vi "sub_statistics.vi"(7 "cmd":enum16{"ini", "read", "write"}(ring), 8 "error in":errorcluster) -> (0 "error out":errorcluster caption="error in")   [LabVIEW 2019]
uses:
  Ctrl/pid-in-params.ctl
  Ctrl/cmd_ini-RW.ctl
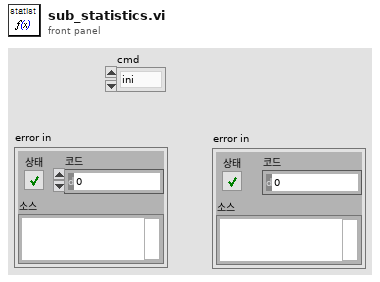
[diagram p1: front panel]
types:
  T1 = typedef "pid-in-params.ctl" = enum16{"read", "write"}
  T2 = typedef "cmd_ini-RW.ctl" = enum16{"ini", "read", "write"}
  T3 = cluster{"deg_agv-lookahead":dbl, "deg_waypoint":dbl, "deg_gap":dbl, "deg_target":dbl, "pid output":dbl, "dis-gap":dbl, "deg_agv-center":dbl}
  T4 = typedef "statistics_val.ctl" = cluster{"gap plus mean":dbl, "gap plus max":dbl, "gap plus sum":dbl, "gap minus mean":dbl, "gap minus max":dbl, "gap minus sum":dbl, "gap abs mean":dbl, "gap abs max":dbl, "gap abs sum":dbl, "wpt length":dbl, "total moving time":dbl, "average speed":dbl, "plus gap count":u64, "minus gap count":u64, "drive length":dbl}
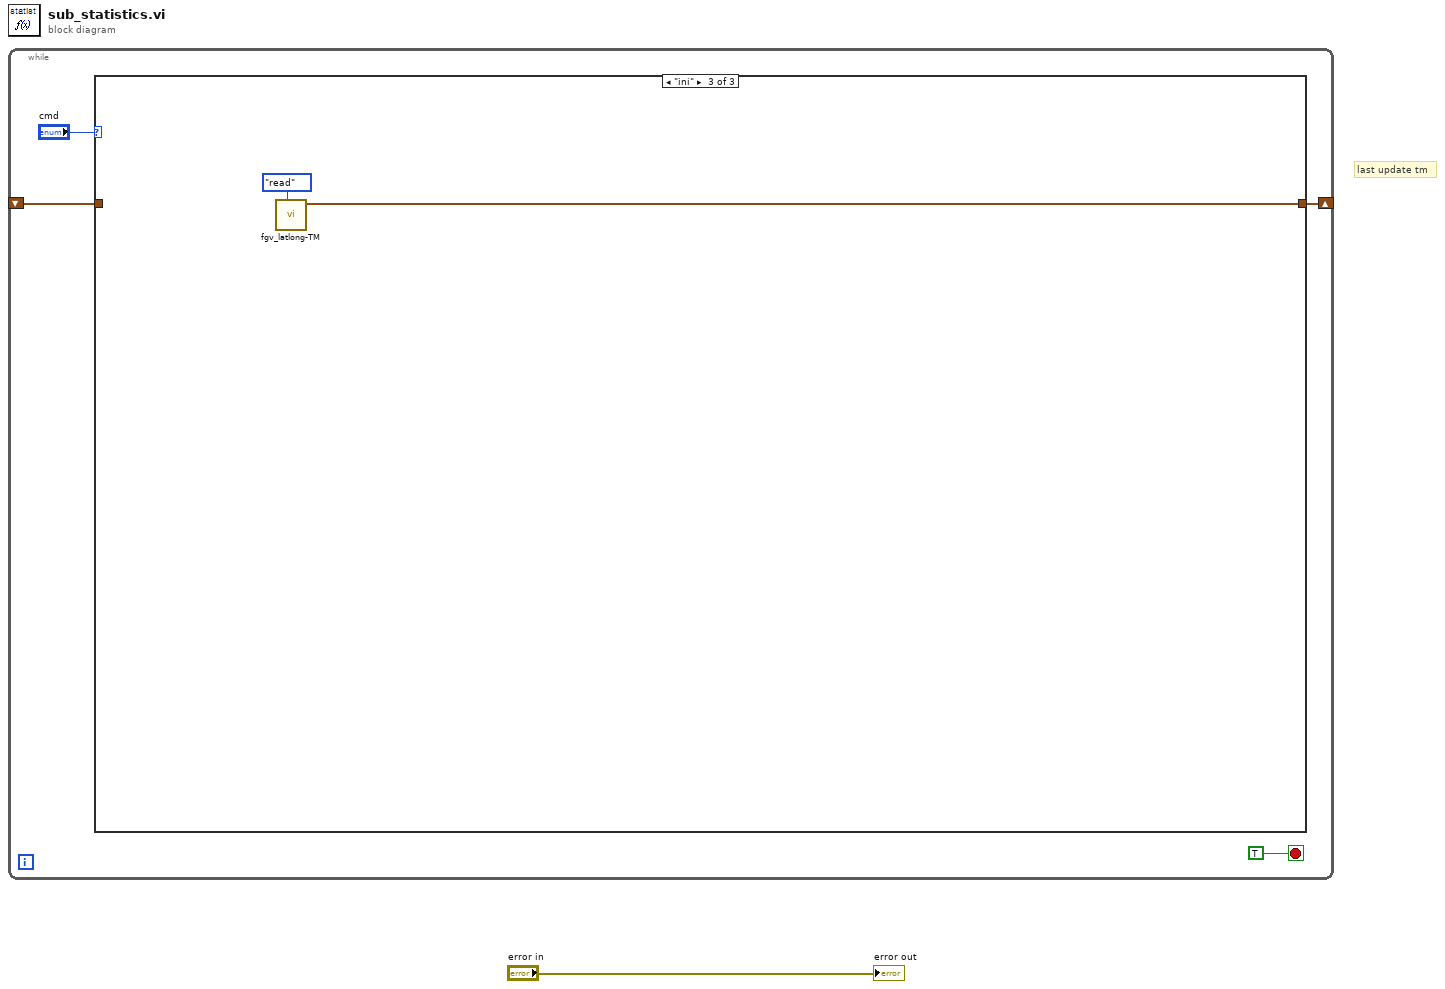
[diagram p0: block diagram]
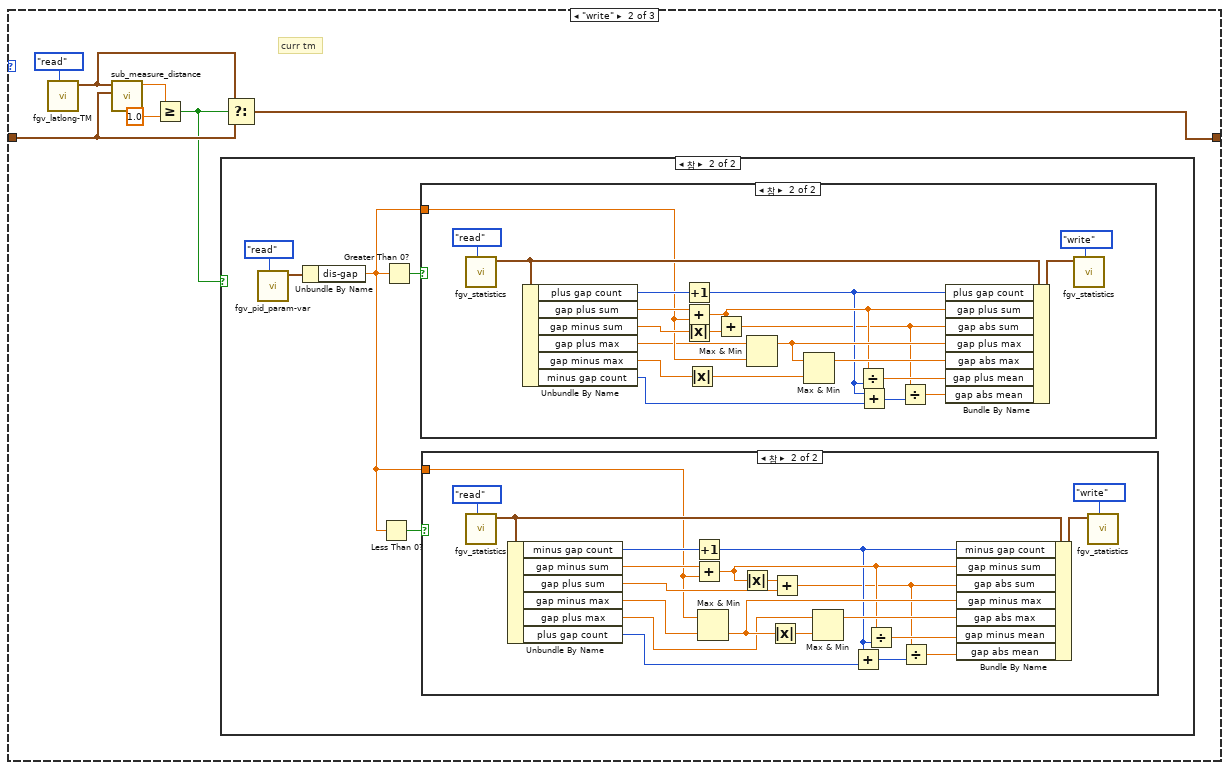
[diagram p3: hidden frame]
diagram:
  # "last update tm"
  n1 = while {
    shift-right: [w3] -> _
    shift-left: _ -> [w2]
    stop <- TRUE stop-if-true
    n2 = case shown="\"ini\"" "cmd" {
      tunnel: [w6 w8 w61] -> w3
      tunnel: w2 -> [w6 w9 _]
      frame "read", Default {
      }
      frame "write" {
        # "curr tm"
        n3 = call "fgv_latlong-TM.vi"("cmd"=enum16{"write", "read"}."read") -> ("tm out"=w10:cluster{dbl, dbl})  [unwired: 9 in, 1 out]
        n4 = call "sub_measure_distance.vi"("pt 2"=w9, "pt 1"=w10) -> ("distance"=w12:dbl)  [unwired: 9 in]
        n5 = Greater Or Equal?(x=w12, y=1.0) -> (x >= y?=w7:bool)
        n6 = case shown="참" w7 {
          frame False {
          }
          frame True {
            n7 = call "fgv_pid_param-var.vi"("cmd"=pid-in-params."read") -> ("pid-var_output"=w17:T3)  [unwired: 10 in]
            n8 = Unbundle By Name(w17) -> ("dis-gap"=w14:dbl)
            n9 = Less Than 0?(x=w14) -> (x < 0?=w15:bool)
            n10 = Greater Than 0?(x=w14) -> (x > 0?=w16:bool)
            n11 = case shown="참" w16 {
              tunnel: w14 -> [_ w52]
              frame False {
              }
              frame True {
                n12 = call "fgv_statistics.vi"("cmd"=cmd_ini-RW."read") -> ("statistics values out"=w59:T4)  [unwired: 10 in]
                n13 = Unbundle By Name(w59) -> ("plus gap count"=w58:u64, "gap plus sum"=w55:dbl, "gap minus sum"=w54:dbl, "gap plus max"=w51:dbl, "gap minus max"=w49:dbl, "minus gap count"=w44:u64)
                n14 = Increment(x=w58) -> (x+1=w43:u64)
                n15 = Add(x=w55, y=w52) -> (x+y=w45:dbl)
                n16 = Absolute Value(x=w54) -> (abs(x)=w53:dbl)
                n17 = Absolute Value(x=w49) -> (abs(x)=w48:dbl)
                n18 = Add(x=w45, y=w53) -> (x+y=w42:dbl)
                n19 = Max & Min(x=w51, y=w52) -> (max(x,y)=w50:dbl)  [unwired: 1 out]
                n20 = Max & Min(x=w50, y=w48) -> (max(x,y)=w47:dbl)  [unwired: 1 out]
                n21 = Divide(x=w45, y=w43) -> (x/y=w46:dbl)
                n22 = Add(x=w43, y=w44) -> (x+y=w41:u64)
                n23 = Divide(x=w42, y=w41) -> (x/y=w40:dbl)
                n24 = Bundle By Name(cluster=w59, "plus gap count"=w43, "gap plus sum"=w45, "gap abs sum"=w42, "gap plus max"=w50, "gap abs max"=w47, "gap plus mean"=w46, "gap abs mean"=w40) -> (w60:T4)
                n25 = call "fgv_statistics.vi"("cmd"=cmd_ini-RW."write", "statistics values"=w60) -> ()  [unwired: 9 in, 1 out]
              }
            }
            n26 = case shown="참" w15 {
              tunnel: w14 -> [_ w32]
              frame False {
              }
              frame True {
                n27 = call "fgv_statistics.vi"("cmd"=cmd_ini-RW."read") -> ("statistics values out"=w38:T4)  [unwired: 10 in]
                n28 = Unbundle By Name(w38) -> ("minus gap count"=w37:u64, "gap minus sum"=w34:dbl, "gap plus sum"=w33:dbl, "gap minus max"=w31:dbl, "gap plus max"=w29:dbl, "plus gap count"=w22:u64)
                n29 = Increment(x=w37) -> (x+1=w23:u64)
                n30 = Add(x=w34, y=w32) -> (x+y=w24:dbl)
                n31 = Max & Min(x=w32, y=w31) -> (min(x,y)=w30:dbl)  [unwired: 1 out]
                n32 = Absolute Value(x=w24) -> (abs(x)=w26:dbl)
                n33 = Absolute Value(x=w30) -> (abs(x)=w28:dbl)
                n34 = Add(x=w26, y=w33) -> (x+y=w21:dbl)
                n35 = Max & Min(x=w29, y=w28) -> (max(x,y)=w27:dbl)  [unwired: 1 out]
                n36 = Add(x=w23, y=w22) -> (x+y=w20:u64)
                n37 = Divide(x=w24, y=w23) -> (x/y=w25:dbl)
                n38 = Divide(x=w21, y=w20) -> (x/y=w19:dbl)
                n39 = Bundle By Name(cluster=w38, "minus gap count"=w23, "gap minus sum"=w24, "gap abs sum"=w21, "gap minus max"=w30, "gap abs max"=w27, "gap minus mean"=w25, "gap abs mean"=w19) -> (w39:T4)
                n40 = call "fgv_statistics.vi"("cmd"=cmd_ini-RW."write", "statistics values"=w39) -> ()  [unwired: 9 in, 1 out]
              }
            }
          }
        }
        n41 = Select(t=w10, s=w7, f=w9) -> (s? t:f=w8:cluster{dbl, dbl})
      }
      frame "ini" {
        n42 = call "fgv_latlong-TM.vi"("cmd"=enum16{"write", "read"}."read") -> ("tm out"=w61:cluster{dbl, dbl})  [unwired: 9 in, 1 out]
      }
    }
  }
  "error out" <- "error in"
